vi "GetCoeffs.vi"(7 "PathToFile":path, 10 "SignalLength":i32, 11 "fs (Hz)":dbl) -> (2 "NyquistLimitedCoefficients":dbl[](array[numeric])=[1.0, 0.9893, 1.019, 1.0269, 1.0344, 1.0416, 1.0487, 1.0558, 1.0628, 1.0701, 1.0776, 1.0854, 1.0937, 1.1026, 1.1121, 1.1224, 1.1336, 1.1457, 1.1589, 1.1733, 1.189, 1.2061, 1.2246, 1.2447, 1.2662, 1.289, 1.3129, 1.3376, 1.3632, 1.3892, 1.4157, 1.4425, 1.4693, 1.496, 1.5226, 1.5491, 1.5754, 1.6016, 1.6277, 1.6535, 1.6792, 1.7046, 1.7298, 1.7548, 1.7794, 1.8033, 1.8263, 1.8483, 1.869, 1.8882, 1.9058, 1.9215, 1.935, 1.9464, 1.9556, 1.9628, 1.9684, 1.9723, 1.9748, 1.9762, 1.9765, 1.9759, 1.9748, 1.9731, 1.9711, 1.9689, 1.9667, 1.9646, 1.9628, 1.9614, 1.9606, 1.9605, 1.9612, 1.963, 1.9657, 1.9693, 1.9738, 1.979, 1.9848, 1.9913, 1.9983, 2.0059, 2.0138, 2.0221, 2.0308, 2.0401, 2.05, 2.0607, 2.0722, 2.0847, 2.0983, 2.113, 0.0, 0.0, 0.0, 0.0, 0.0, 0.0, 0.0, 0.0, 0.0, 0.0, 0.0, 0.0, 0.0, 0.0, 0.0, 0.0, 0.0, 0.0, 0.0, 0.0, 0.0, 0.0, 0.0, 0.0, 0.0, 0.0, 0.0, 0.0, 0.0, 0.0, 0.0, 0.0, 0.0, 0.0, 0.0, 0.0, 0.0, 0.0, 0.0, 0.0, 0.0, 0.0, 0.0, 0.0, 0.0, 0.0, 0.0, 0.0, 0.0, 0.0, 0.0, 0.0])   [LabVIEW 2011]
uses:
  CPP_TubingCompensation/CPP_TubingCompGlobal.vi
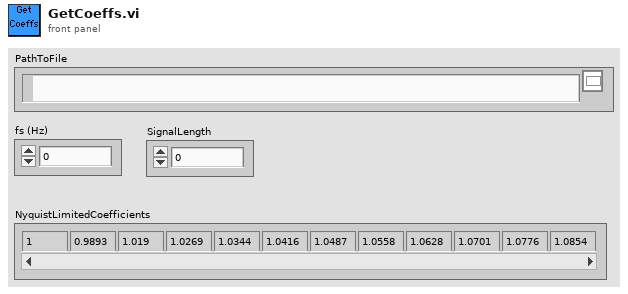
[diagram p1: front panel]
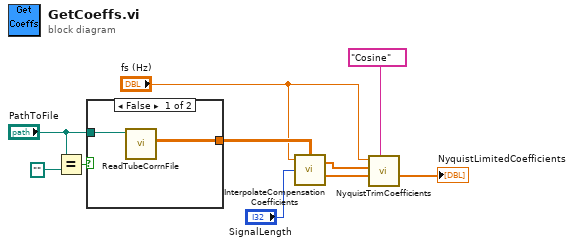
[diagram p0: block diagram]
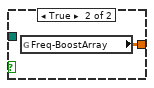
[diagram p2: hidden frame]
diagram:
  n1 = Equal?(x="PathToFile", y=path "") -> (x = y?=w2:bool)
  n2 = case shown="False" w2 {
    tunnel: [w12 w13] -> w10
    tunnel: "PathToFile" -> [w11 _]
    frame False {
      n3 = call "ReadTubeCorrnFile.vi"("PathToFile"=w11) -> ("F-CompArray"=w12:dbl[][])  [unwired: 10 in]
    }
    frame True {
      n4 = global read "CPP_TubingCompGlobal.vi" "Freq-BoostArray"() -> (w13:dbl[][])
    }
  }
  n5 = call "InterpolateCompensationCoefficients.vi"("F-CompArray"=w10, "SignalLength"="SignalLength", "fs (Hz)"="fs (Hz)") -> ("InterpolatedCoefficients"=w8:dbl[], "Frequencies"=w9:dbl[])  [unwired: 1 in]
  n6 = call "NyquistTrimCoefficients.vi"("Cutoff type"="Cosine", "InterpolatedCoefficients"=w8, "Frequencies"=w9, "fs (Hz)"="fs (Hz)") -> ("NyquistLimitedCoefficients"=→"NyquistLimitedCoefficients":dbl[])  [unwired: 6 in, 1 out]
